vi "GUID Generator.vi"() -> ()   [LabVIEW 2018]
panel:
  in  "Write GUID to Clipboard?":bool=TRUE
  out "GUID":string
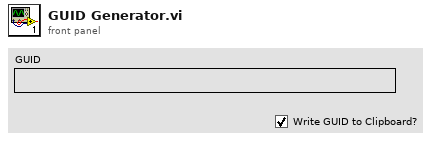
[diagram p1: front panel]
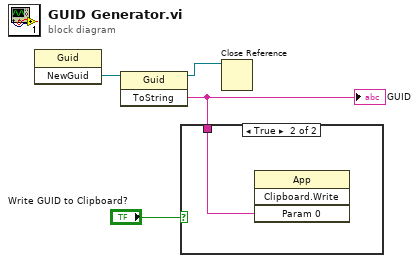
[diagram p0: block diagram]
diagram:
  n1 = invoke class="Guid" method="NewGuid"() -> ("NewGuid"=w4:refnum<k24>)  [unwired: 3 in, 2 out]
  n2 = invoke class="Guid" method="ToString"(reference=w4) -> (reference out=w3:refnum<k24>, "ToString"=w1:string)  [unwired: 2 in, 1 out]
  "GUID" <- w1
  n3 = case shown="True" "Write GUID to Clipboard?" {
    tunnel: w1 -> [_ w5]
    frame False {
    }
    frame True {
      n4 = invoke class="App" method="Clipboard.Write"("Param 0"=w5) -> ()  [unwired: 3 in, 4 out]
    }
  }
  n5 = Close Reference(reference=w3) -> ()  [unwired: 1 in, 1 out]
